vi "Create and Read DO.vi"(8 "error in":errorcluster, 10 "initial channel settings":T1[](array[typedef]), 11 "NI 9475 Test in":refnum<class "NI 9482 Test.lvclass">) -> (0 "error out":errorcluster, 2 "read channel settings":T1[](array[typedef]), 3 "NI 9475 Test out":refnum<class "NI 9482 Test.lvclass">)   [LabVIEW 2017, in "NI 9482 Test.lvclass"]
uses:
  NI 9482 Test.lvclass
  Scripting/Modules/NI 9482/NI 9482.lvclass
  Scripting/Modules/Mode Classes/Controls/digital channel settings.ctl
  Scripting/Scan Engine Scripting.lvlib
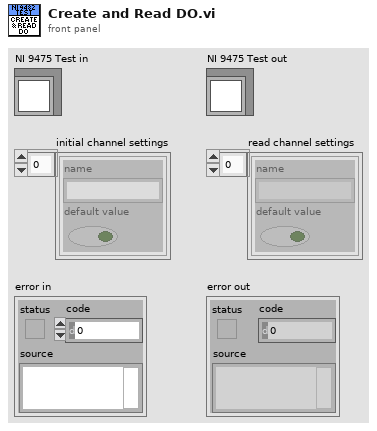
[diagram p1: front panel]
types:
  T1 = typedef "Scan Engine Scripting.lvlib/digital channel settings.ctl" = cluster{"name":string, "default value":bool}
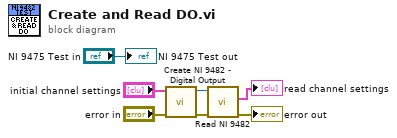
[diagram p0: block diagram]
diagram:
  n1 = call "Create NI 9482 - Digital Output.vi"("error in"="error in", "channel settings"="initial channel settings") -> ("error out"=w7:errorcluster, "NI 9482 out"=w4:refnum<class "NI 9482.lvclass">)  [unwired: 8 in]
  n2 = call "Read NI 9482.vi"("error in"=w7, "NI 9482 in"=w4) -> ("error out"=→"error out":errorcluster, "channel settings"=→"read channel settings":T1[])  [unwired: 7 in, 1 out]
  "NI 9475 Test out" <- "NI 9475 Test in"
